vi "Coerce Duty Cycle.vi"(0 "duty cycle (scaled) in":u32, 7 "frequency (scaled)":u32, 11 "error in (no error)":errorcluster) -> (4 "duty cycle (scaled) out":u32, 15 "error out":errorcluster)   [LabVIEW 2020, in "NI_FpgaMspHost.lvlib"]
doc: "Limits range and resolution of non-zero duty cycles requestable for a given frequency by taking into account the sample period implied by <B>frequency (scaled)</B>."
uses:
  <vilib>/rvi/Analysis/host/Public/NI_FpgaMspHost.lvlib
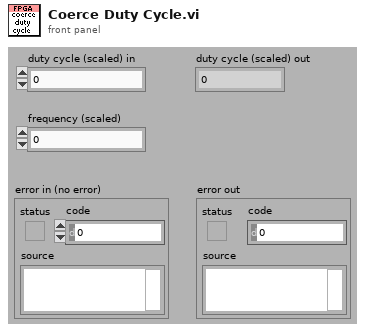
[diagram p1: front panel]
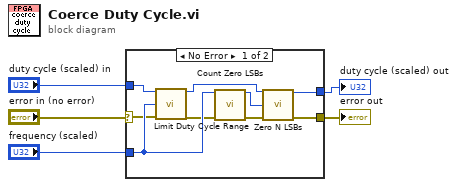
[diagram p0: block diagram]
diagram:
  n1 = case shown="No Error" "error in (no error)" {
    selector: "error in (no error)" -> [w6 w16]
    tunnel: [w9 w15] -> w5
    tunnel: "duty cycle (scaled) in" -> [w12 w15]
    tunnel: "frequency (scaled)" -> [w13 _]
    tunnel: [w14 w16] -> w2
    frame No Error {
      n2 = call <vilib>:"Limit Duty Cycle Range.vi"("duty cycle (scaled) in"=w12, "frequency (scaled)"=w13, "error in (no error)"=w6) -> ("duty cycle (scaled) out"=w11:u32, "error out"=w8:errorcluster)  [unwired: 2 in, 9 out]
      n3 = call <vilib>:"Count Zero LSBs.vi"("input"=w13, "error in (no error)"=w8) -> ("trailing zeros"=w10:i32, "error out"=w7:errorcluster)  [unwired: 2 in, 10 out]
      n4 = call <vilib>:"Zero N LSBs.vi"("input"=w11, "N"=w10, "error in (no error)"=w7) -> ("quantized output"=w9:u32, "error out"=w14:errorcluster)  [unwired: 2 in, 9 out]
    }
    frame Error {
    }
  }
  "duty cycle (scaled) out" <- w5
  "error out" <- w2
